vi "__SIS_Heat_Set.vi"(7 "Heat_VoltegeiVj":dbl=24.0, 9 "Set_Heat_state(0:OFF 1:ON)":u8, 10 "Bias_LO_equip":T1={"Node address"=19, "CAN Interface"="CAN0", "Cartridge band"=10, "Slave Node in"={"Address"=19, "Serial Number"=[16, 71, 55, 76, 1, 8, 0, -15]}, "ObjHandle out"=89653312, "POL"=1, "sb"=1, "GPIB_SM (SIS S,V)"="24", "GPIB_DMM (SIS I)"="22", "GPIB_SM (MAG I) "="25", "GPIB_SG(LO)"="19", "GPIB_PW (PAMP) "="6", "GPIB_TMP1(8ch)"="12", "GPIB_TMP2(2ch)  "="13", "WCA_avg"=10, "Rsen"=10.0, "BiasModule"=0, "LOModule "=1, "WCA_LO_FREQ_SET"={"YTO Low freq. [GHz]"=14.42, "YTO High freq. [GHz]"=17.7, "Kvco"=1, "Lock Pol."=0, "SET LO FREQ"=72.5, "Multiplier"=6.0, "YTO (HEX)"=0, "YTO coarse( FREQ)"=25.0, "NULL PLL INTEGRATOR"=FALSE}, "Res for"=0} {"Res for" items=["none", "series res", "parallel res"]; "WCA_LO_FREQ_SET"."YTO coarse( FREQ)" min=25 max=150 step=0.0001 format="%.3f"; "WCA_LO_FREQ_SET"."Multiplier" min=3 max=6 step=3; "WCA_LO_FREQ_SET"."SET LO FREQ" min=25 max=150 step=0.0001 format="%.3f"; "WCA_LO_FREQ_SET"."Lock Pol." items=["Lower", "Upper"]; "WCA_LO_FREQ_SET"."Kvco" items=["7.5MHz/V", "15MHz/V"]; "WCA_LO_FREQ_SET"."YTO High freq. [GHz]" format="%.3f"; "WCA_LO_FREQ_SET"."YTO Low freq. [GHz]" format="%.3f"; "LOModule" items=["Manual", "B10Lab LO", "WCA LO"]; "BiasModule" items=["B10Lab Bias", "WCA BiasModule"]; "Slave Node in"."Serial Number" format="%.0x"; "Slave Node in"."Address" format="%.0x"; "Cartridge band" max=10 step=1; "Node address" format="%.0x"}, 11 "GPIB_PW (SISHeater)":string="3") -> (2 "“d—¬":dbl)   [LabVIEW 2017]
panel:
  # "LO freq. [GHz]"
  # "YTO LOW\n/High Freq."
  # "ZERO Intgrtr"
  # "Node Address"
  # "Serial Number"
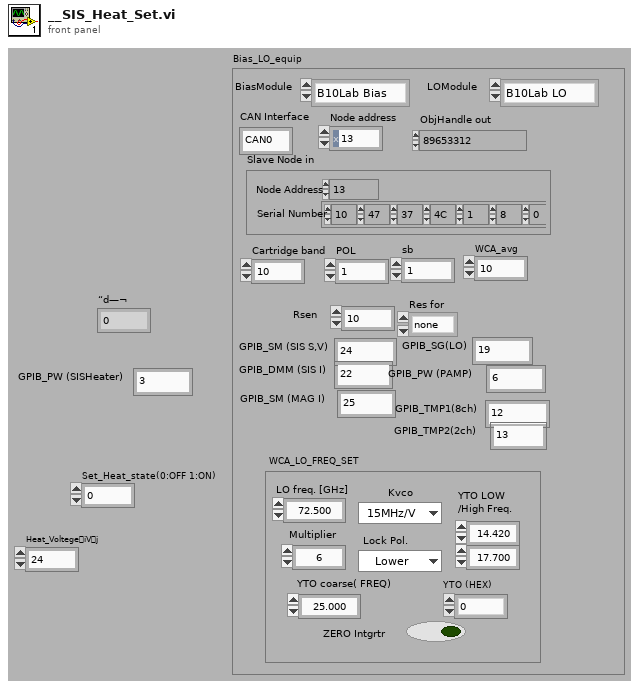
[diagram p1: front panel]
types:
  T1 = cluster{"Node address":u16, "CAN Interface":string, "Cartridge band":u32, "Slave Node in":cluster{"Address":i16, "Serial Number":i8[]}, "ObjHandle out":u32, "POL":u32, "sb":u32, "GPIB_SM (SIS S,V)":string, "GPIB_DMM (SIS I)":string, "GPIB_SM (MAG I) ":string, "GPIB_SG(LO)":string, "GPIB_PW (PAMP) ":string, "GPIB_TMP1(8ch)":string, "GPIB_TMP2(2ch)  ":string, "WCA_avg":i32, "Rsen":dbl, "BiasModule":u16, "LOModule ":u16, "WCA_LO_FREQ_SET":cluster{"YTO Low freq. [GHz]":sgl, "YTO High freq. [GHz]":sgl, "Kvco":u16, "Lock Pol.":u16, "SET LO FREQ":sgl, "Multiplier":sgl, "YTO (HEX)":u16, "YTO coarse( FREQ)":sgl, "NULL PLL INTEGRATOR":bool}, "Res for":u16}
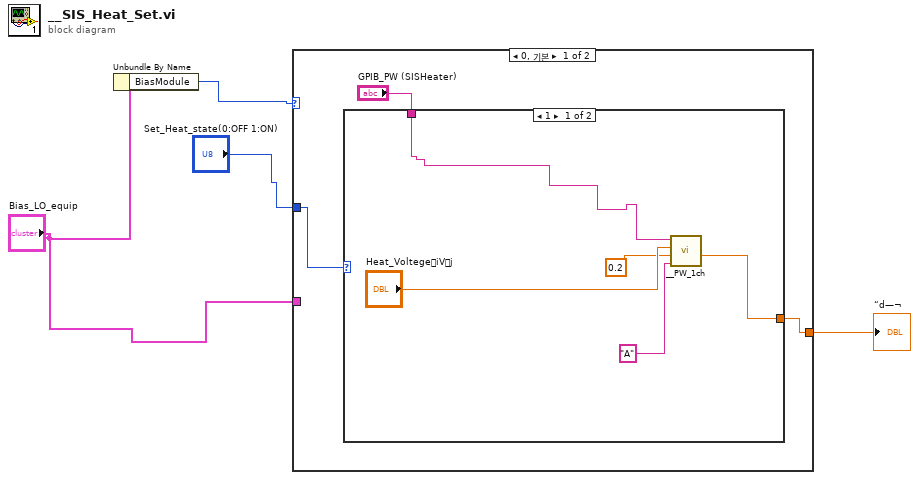
[diagram p0: block diagram]
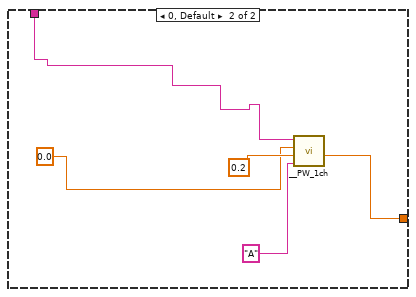
[diagram p2: hidden frame]
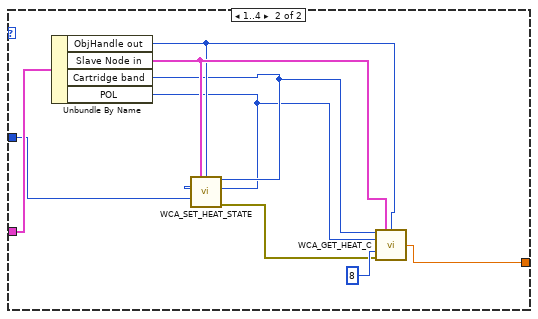
[diagram p3: hidden frame]
diagram:
  n1 = Unbundle By Name("Bias_LO_equip") -> ("BiasModule"=w2:u16)
  n2 = case shown="0, 기본" w2 {
    tunnel: "Bias_LO_equip" -> [_ w26]
    tunnel: "Set_Heat_state(0:OFF 1:ON)" -> [w6 w25]
    tunnel: [w7 w18] -> w1
    frame 0, Default {
      n3 = case shown="1" w6 {
        tunnel: [w9 w15] -> w7
        tunnel: "GPIB_PW (SISHeater)" -> [w8 w13]
        frame 1 {
          n4 = call "__PW_1ch.vi"("ChiA,B,C,Dj"="A", "A(A)"=0.2, "V(V)"="Heat_VoltegeiVj", "GPIB"=w8) -> ("Amoni"=w9:dbl)  [unwired: 6 in, 1 out]
        }
        frame 0, Default {
          n5 = call "__PW_1ch.vi"("ChiA,B,C,Dj"="A", "A(A)"=0.2, "V(V)"=0.0, "GPIB"=w13) -> ("Amoni"=w15:dbl)  [unwired: 6 in, 1 out]
        }
      }
    }
    frame 1..4 {
      n6 = Unbundle By Name(w26) -> ("ObjHandle out"=w23:u32, "Slave Node in"=w24:cluster{"Address":i16, "Serial Number":i8[]}, "Cartridge band"=w22:u32, "POL"=w21:u32)
      n7 = call "WCA_SET_HEAT_STATE.vi"("Cartridge Band"=w22, "Slave Node in"=w24, "ObjHandle in"=w23, "POL"=w21, "SET_MIX_HEAT_STATE"=w25) -> ("error out"=w19:errorcluster)  [unwired: 9 in, 1 out]
      n8 = call "WCA_GET_HEAT_C.vi"("Cartridge Band"=w22, "Slave Node in"=w24, "ObjHandle in"=w23, "POL"=w21, "avg"=8, "error in (no error)"=w19) -> ("get"=w18:dbl)  [unwired: 7 in, 2 out]
    }
  }
  "“d—¬" <- w1
